vi "Get Settings ID (Group).vi"(8 "error in (no error)":errorcluster, 11 "Item Ref in":T2 format="%.0x") -> (0 "error out":errorcluster, 2 "settings id":T1={"plugin"=-1, "thread"=-1, "group"=-1, "transfer"=-1, "channel"=-1}, 3 "Item Ref out":T2 format="%.0x")   [LabVIEW 2017, in "DSF System Explorer.lvlib"]
uses:
  DSF System Explorer.lvlib
  <vilib>/NI Veristand/Custom Device API/Custom Device Item Ref.ctl
  DSF Core.lvlibp/Typedefs/DSF Configuration ID.ctl
  <vilib>/NI Veristand/Custom Device API/Custom Device API.lvlib
  DSF Core.lvlibp
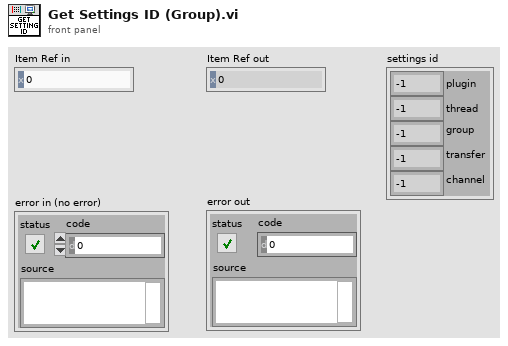
[diagram p1: front panel]
types:
  T1 = typedef "DSF Core.lvlibp/DSF Configuration ID.ctl" = cluster{"plugin":i32, "thread":i32, "group":i32, "transfer":i32, "channel":i32}
  T2 = typedef "Custom Device API.lvlib/Custom Device Item Ref.ctl" = u64
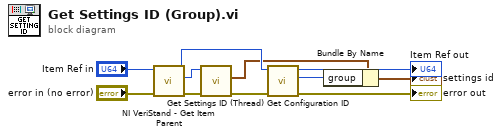
[diagram p0: block diagram]
diagram:
  n1 = call <vilib>:"NI VeriStand - Get Item Parent.vi"("error in (no error)"="error in (no error)", "Item Ref in"="Item Ref in") -> ("error out"=w4:errorcluster, "Parent Ref"=w3:T2, "Item Ref out"=w5:T2)  [unwired: 6 in, 1 out]
  n2 = call "Get Settings ID (Thread).vi"("error in (no error)"=w4, "Item Ref in"=w3) -> ("error out"=w2:errorcluster, "settings id"=w1:T1)  [unwired: 7 in, 1 out]
  n3 = call "Get Configuration ID.vi"("error in (no error)"=w2, "Item Ref in"=w5) -> ("error out"=→"error out":errorcluster, "Configuration ID"=w11:i32, "Item Ref out"=→"Item Ref out":T2)  [unwired: 7 in]
  n4 = Bundle By Name(cluster=w1, "group"=w11) -> (→"settings id":T1)
